vi "Calculate Place points.vi"(8 "error in (no error)":errorcluster, 11 "Control in":refnum<class "Control.lvclass">) -> (0 "error out":errorcluster, 3 "Control out":refnum<class "Control.lvclass">)   [LabVIEW 2012, in "Control.lvclass"]
uses:
  Control.lvclass
  Control.lvclass/Control.ctl
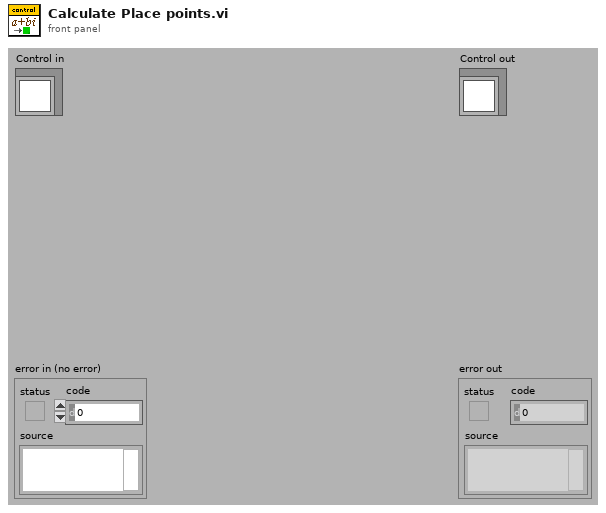
[diagram p1: front panel]
types:
  T1 = enum16{"User-specified Font", "Application Font", "System Font", "Dialog Font"}
  T2 = typedef "Control.lvclass/BX.Orientation__LCR _Modified.ctl" = u8
  T3 = typedef "Control.lvclass/_ui_tools_font.ctl" = cluster{"Font Name:":string, "Size":i16, "Strikeout?":bool, "Italic?":bool, "Underline?":bool, "Outline?":bool, "Shadow?":bool, "Bold?":bool}
  T4 = cluster{"left":i16, "top":i16, "right":i16, "bottom":i16}
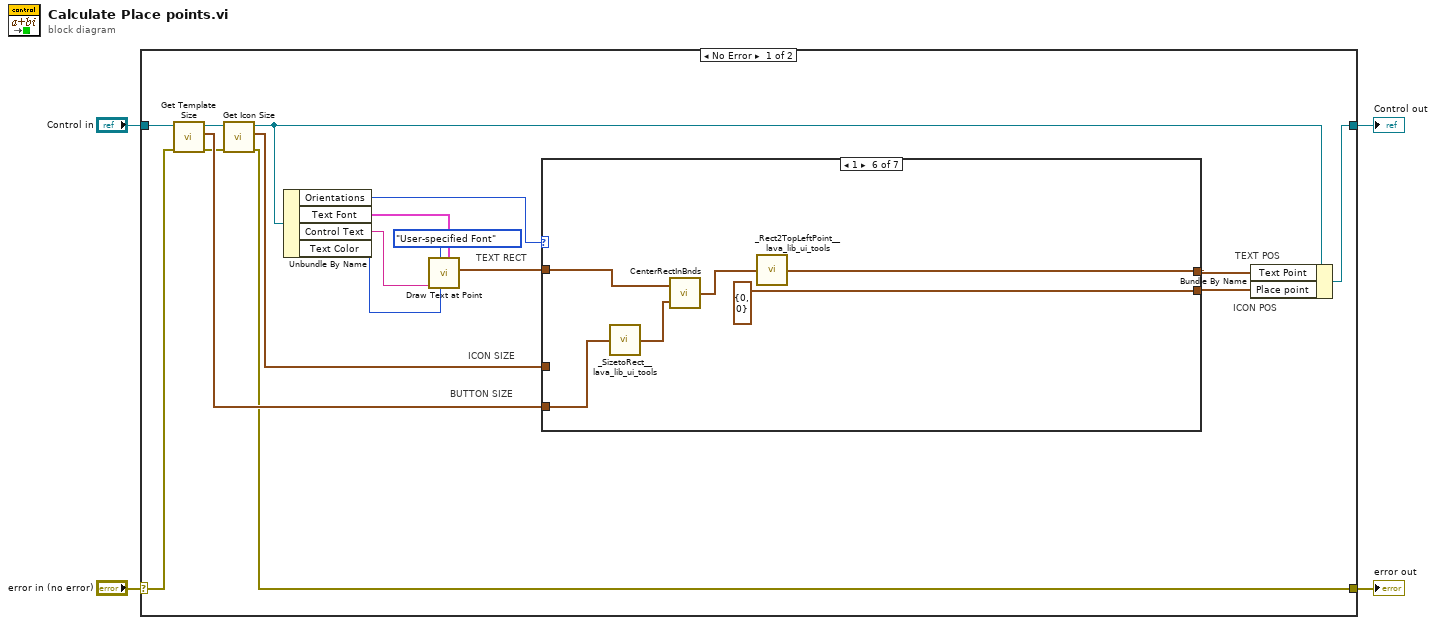
[diagram p0: block diagram]
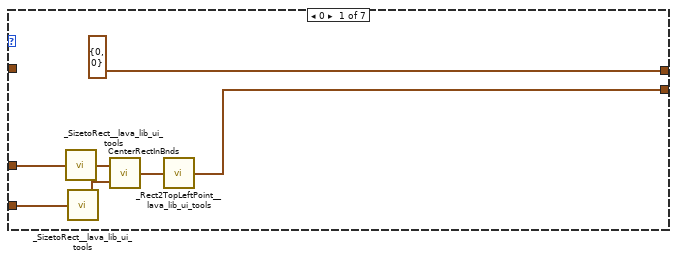
[diagram p2: hidden frame]
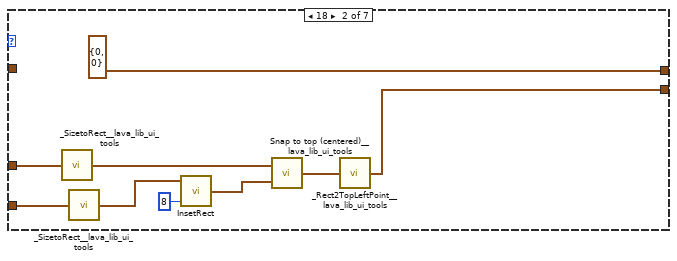
[diagram p3: hidden frame]
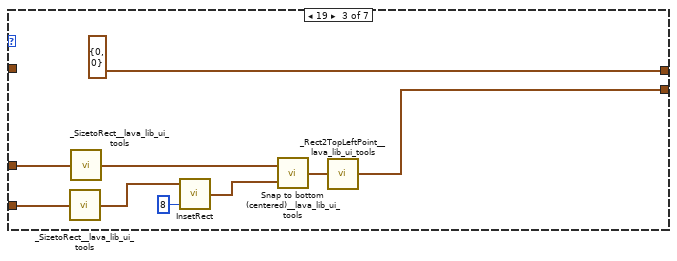
[diagram p4: hidden frame]
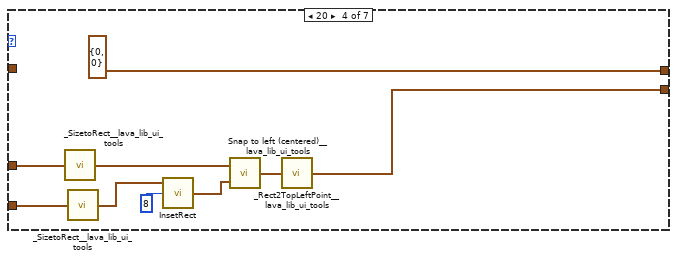
[diagram p5: hidden frame]
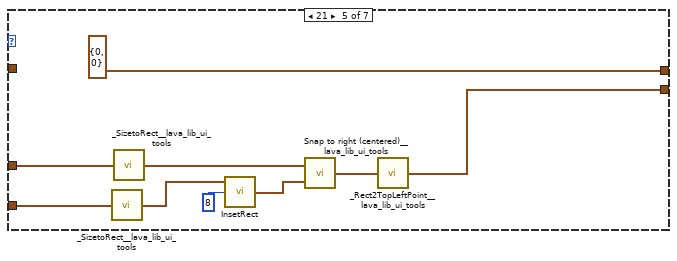
[diagram p6: hidden frame]
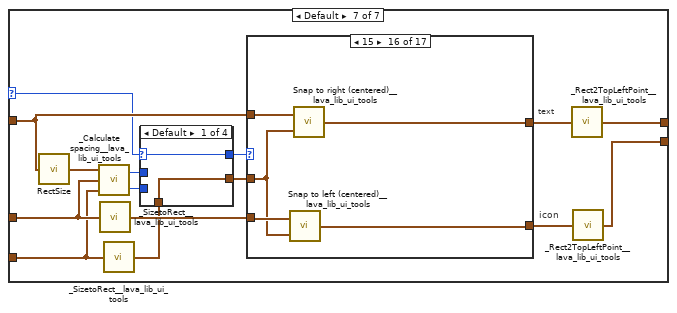
[diagram p7: hidden frame]
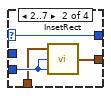
[diagram p8: hidden frame]
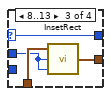
[diagram p9: hidden frame]
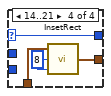
[diagram p10: hidden frame]
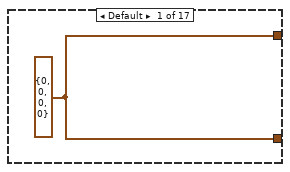
[diagram p11: hidden frame]
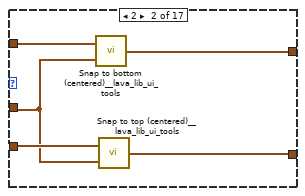
[diagram p12: hidden frame]
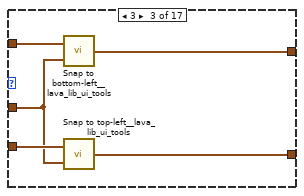
[diagram p13: hidden frame]
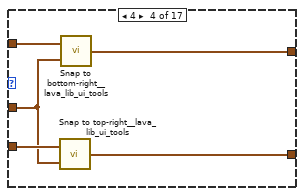
[diagram p14: hidden frame]
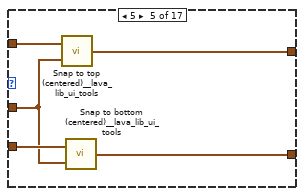
[diagram p15: hidden frame]
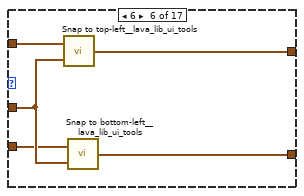
[diagram p16: hidden frame]
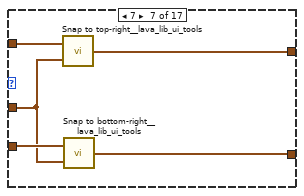
[diagram p17: hidden frame]
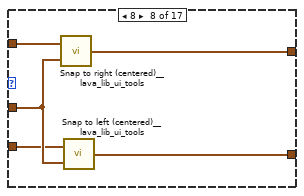
[diagram p18: hidden frame]
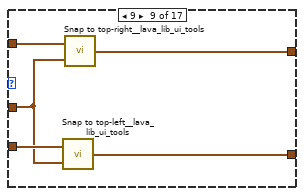
[diagram p19: hidden frame]
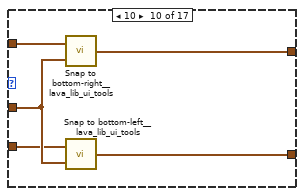
[diagram p20: hidden frame]
diagram:
  n1 = case shown="No Error" "error in (no error)" {
    selector: "error in (no error)" -> [w15 w197]
    tunnel: [w6 w197] -> w3
    tunnel: [w9 w196] -> w1
    tunnel: "Control in" -> [w14 w196]
    frame No Error {
      # "TEXT RECT"
      # "ICON SIZE"
      # "BUTTON SIZE"
      # "TEXT POS"
      # "ICON POS"
      n2 = call-dynamic "Get Template Size.vi"("error in (no error)"=w15, "Control in"=w14) -> ("error out"=w16:errorcluster, "Button Size"=w18:cluster{"Width":i32, "Height":i32}, "Control out"=w21:refnum<class "Control.lvclass">)  [unwired: 7 out]
      n3 = call-dynamic "Get Icon Size.vi"("error in (no error)"=w16, "Control in"=w21) -> ("error out"=w6:errorcluster, "Icon Size"=w19:cluster{"Width":i32, "Height":i32}, "Control out"=w10:refnum<class "Control.lvclass">)  [unwired: 7 out]
      n4 = Unbundle By Name(w10) -> ("Orientations"=w11:T2, "Text Font"=w12:T3, "Control Text"=w13:string, "Text Color"=w5:u32)
      n5 = call <vilib>:"Draw Text at Point.vi"("[user-specified font]"=w12, "text color(black)"=w5, "desired font(Application)"=T1."User-specified Font", "text"=w13) -> ("text rect"=w17:T4)  [unwired: 5 in, 2 out]
      n6 = case shown="1" w11 {
        selector: w11 -> [_ _ _ _ _ _ w75]
        tunnel: [cluster{"x":i32, "y":i32} {"x"=0, "y"=0} ("Point") cluster{"x":i32, "y":i32} {"x"=0, "y"=0} ("Point") cluster{"x":i32, "y":i32} {"x"=0, "y"=0} ("Point") cluster{"x":i32, "y":i32} {"x"=0, "y"=0} ("Point") cluster{"x":i32, "y":i32} {"x"=0, "y"=0} ("Point") w65 w85] -> w8
        tunnel: [w22 w32 w41 w50 w57 cluster{"x":i32, "y":i32} {"x"=0, "y"=0} ("Point") w82] -> w7
        tunnel: w18 -> [w26 w33 w43 w48 w61 w68 w72]
        tunnel: w17 -> [_ _ _ _ _ w70 w78]
        tunnel: w19 -> [w24 w35 w44 w52 w62 _ w83]
        frame 0 {
          n7 = call <vilib>:"_SizetoRect__lava_lib_ui_tools.vi"("size"=w24) -> ("bounds"=w25:T4)  [unwired: 4 out]
          n8 = call <vilib>:"_SizetoRect__lava_lib_ui_tools.vi"("size"=w26) -> ("bounds"=w27:T4)  [unwired: 4 out]
          n9 = call <vilib>:"CenterRectInBnds.vi"("bounds"=w27, "rect"=w25) -> ("centered rect"=w23:T4)
          n10 = call <vilib>:"_Rect2TopLeftPoint__lava_lib_ui_tools.vi"("bounds"=w23) -> ("TopLeft point"=w22:cluster{"x":i32, "y":i32})  [unwired: 4 out]
        }
        frame 18 {
          n11 = call <vilib>:"_SizetoRect__lava_lib_ui_tools.vi"("size"=w35) -> ("bounds"=w31:T4)  [unwired: 4 out]
          n12 = call <vilib>:"_SizetoRect__lava_lib_ui_tools.vi"("size"=w33) -> ("bounds"=w34:T4)  [unwired: 4 out]
          n13 = call <vilib>:"InsetRect.vi"("dv"=i16 8 ("dh"), "rect"=w34) -> ("inset rect"=w30:T4)  [unwired: 1 in]
          n14 = call <vilib>:"Snap to top (centered)__lava_lib_ui_tools.vi"("Large Rect"=w30, "Small Rect"=w31) -> ("Snapped to top center"=w29:T4)
          n15 = call <vilib>:"_Rect2TopLeftPoint__lava_lib_ui_tools.vi"("bounds"=w29) -> ("TopLeft point"=w32:cluster{"x":i32, "y":i32})  [unwired: 4 out]
        }
        frame 19 {
          n16 = call <vilib>:"_SizetoRect__lava_lib_ui_tools.vi"("size"=w43) -> ("bounds"=w42:T4)  [unwired: 4 out]
          n17 = call <vilib>:"_SizetoRect__lava_lib_ui_tools.vi"("size"=w44) -> ("bounds"=w40:T4)  [unwired: 4 out]
          n18 = call <vilib>:"InsetRect.vi"("dv"=i16 8 ("dh"), "rect"=w42) -> ("inset rect"=w39:T4)  [unwired: 1 in]
          n19 = call <vilib>:"Snap to bottom (centered)__lava_lib_ui_tools.vi"("Large Rect"=w39, "Small Rect"=w40) -> ("Snapped to bottom center"=w38:T4)
          n20 = call <vilib>:"_Rect2TopLeftPoint__lava_lib_ui_tools.vi"("bounds"=w38) -> ("TopLeft point"=w41:cluster{"x":i32, "y":i32})  [unwired: 4 out]
        }
        frame 20 {
          n21 = call <vilib>:"_SizetoRect__lava_lib_ui_tools.vi"("size"=w52) -> ("bounds"=w53:T4)  [unwired: 4 out]
          n22 = call <vilib>:"_SizetoRect__lava_lib_ui_tools.vi"("size"=w48) -> ("bounds"=w47:T4)  [unwired: 4 out]
          n23 = call <vilib>:"InsetRect.vi"("dh"=i16 8, "rect"=w47) -> ("inset rect"=w49:T4)  [unwired: 1 in]
          n24 = call <vilib>:"Snap to left (centered)__lava_lib_ui_tools.vi"("Large Rect"=w49, "Small Rect"=w53) -> ("Snapped to left center"=w51:T4)
          n25 = call <vilib>:"_Rect2TopLeftPoint__lava_lib_ui_tools.vi"("bounds"=w51) -> ("TopLeft point"=w50:cluster{"x":i32, "y":i32})  [unwired: 4 out]
        }
        frame 21 {
          n26 = call <vilib>:"_SizetoRect__lava_lib_ui_tools.vi"("size"=w61) -> ("bounds"=w60:T4)  [unwired: 4 out]
          n27 = call <vilib>:"_SizetoRect__lava_lib_ui_tools.vi"("size"=w62) -> ("bounds"=w59:T4)  [unwired: 4 out]
          n28 = call <vilib>:"InsetRect.vi"("dh"=i16 8, "rect"=w60) -> ("inset rect"=w58:T4)  [unwired: 1 in]
          n29 = call <vilib>:"Snap to right (centered)__lava_lib_ui_tools.vi"("Large Rect"=w58, "Small Rect"=w59) -> ("Snapped to right center"=w56:T4)
          n30 = call <vilib>:"_Rect2TopLeftPoint__lava_lib_ui_tools.vi"("bounds"=w56) -> ("TopLeft point"=w57:cluster{"x":i32, "y":i32})  [unwired: 4 out]
        }
        frame 1 {
          n31 = call <vilib>:"_SizetoRect__lava_lib_ui_tools.vi"("size"=w68) -> ("bounds"=w67:T4)  [unwired: 4 out]
          n32 = call <vilib>:"CenterRectInBnds.vi"("bounds"=w67, "rect"=w70) -> ("centered rect"=w66:T4)
          n33 = call <vilib>:"_Rect2TopLeftPoint__lava_lib_ui_tools.vi"("bounds"=w66) -> ("TopLeft point"=w65:cluster{"x":i32, "y":i32})  [unwired: 4 out]
        }
        frame Default {
          # "icon"
          # "text"
          n34 = call <vilib>:"RectSize.vi"("rect"=w78) -> ("point"=w84:cluster{"x":i16, "y":i16})
          n35 = call <vilib>:"_Calculate spacing__lava_lib_ui_tools.vi"("Button Size"=w72, "Icon Size"=w83, "Text Size"=w84) -> ("Vert. spacing"=w81:i32, "Horiz. spacing"=w74:i32)
          n36 = call <vilib>:"_SizetoRect__lava_lib_ui_tools.vi"("size"=w83) -> ("bounds"=w80:T4)  [unwired: 4 out]
          n37 = call <vilib>:"_SizetoRect__lava_lib_ui_tools.vi"("size"=w72) -> ("bounds"=w71:T4)  [unwired: 4 out]
          n38 = case shown="Default" w75 {
            selector: w75 -> [w86 w88 w92 w97]
            tunnel: w81 -> [_ w91 _ _]
            tunnel: [w87 w90 w95 w99] -> w77
            tunnel: w71 -> [w87 w89 w94 w98]
            tunnel: w74 -> [_ _ w93 _]
            tunnel: [w86 w88 w92 w97] -> w73
            frame Default {
            }
            frame 2..7 {
              n39 = call <vilib>:"InsetRect.vi"("dv"=w91, "dh"=w91, "rect"=w89) -> ("inset rect"=w90:T4)
            }
            frame 8..13 {
              n40 = call <vilib>:"InsetRect.vi"("dv"=w93, "dh"=w93, "rect"=w94) -> ("inset rect"=w95:T4)
            }
            frame 14..21 {
              w96 = i16 8 ("dh")
              n41 = call <vilib>:"InsetRect.vi"("dv"=w96, "dh"=w96, "rect"=w98) -> ("inset rect"=w99:T4)
            }
          }
          n42 = case shown="15" w73 {
            tunnel: w80 -> [_ w103 w108 w115 w119 w123 w128 w132 w139 w142 w148 w154 w157 w172 w178 w190 w192]
            tunnel: [w100 w101 w106 w114 w120 w122 w129 w131 w136 w141 w146 w155 w158 w167 w177 w189 w193] -> w79
            tunnel: w78 -> [_ w105 w110 w112 w118 w125 w126 w135 w140 w144 w150 w153 w159 w171 w176 w188 w195]
            tunnel: w77 -> [_ w102 w107 w113 w117 w124 w127 w133 w138 w145 w147 w152 w156 w170 w175 w187 w191]
            tunnel: [w100 w104 w109 w111 w116 w121 w130 w134 w137 w143 w149 w151 w160 w168 w185 w186 w194] -> w76
            frame Default {
              w100 = T4 {"left"=0, "top"=0, "right"=0, "bottom"=0} ("Snapped to bottom left")
            }
            frame 2 {
              n43 = call <vilib>:"Snap to bottom (centered)__lava_lib_ui_tools.vi"("Large Rect"=w102, "Small Rect"=w105) -> ("Snapped to bottom center"=w104:T4)
              n44 = call <vilib>:"Snap to top (centered)__lava_lib_ui_tools.vi"("Large Rect"=w102, "Small Rect"=w103) -> ("Snapped to top center"=w101:T4)
            }
            frame 3 {
              n45 = call <vilib>:"Snap to bottom-left__lava_lib_ui_tools.vi"("Fixed Rect"=w107, "Rect"=w110) -> ("Snapped to bottom left"=w109:T4)
              n46 = call <vilib>:"Snap to top-left__lava_lib_ui_tools.vi"("Fixed Rect"=w107, "Rect"=w108) -> ("Snapped to top left"=w106:T4)
            }
            frame 4 {
              n47 = call <vilib>:"Snap to top-right__lava_lib_ui_tools.vi"("Fixed Rect"=w113, "Rect"=w115) -> ("Snapped to top left"=w114:T4)
              n48 = call <vilib>:"Snap to bottom-right__lava_lib_ui_tools.vi"("Fixed Rect"=w113, "Rect"=w112) -> ("Snapped to bottom right"=w111:T4)
            }
            frame 5 {
              n49 = call <vilib>:"Snap to top (centered)__lava_lib_ui_tools.vi"("Large Rect"=w117, "Small Rect"=w118) -> ("Snapped to top center"=w116:T4)
              n50 = call <vilib>:"Snap to bottom (centered)__lava_lib_ui_tools.vi"("Large Rect"=w117, "Small Rect"=w119) -> ("Snapped to bottom center"=w120:T4)
            }
            frame 6 {
              n51 = call <vilib>:"Snap to top-left__lava_lib_ui_tools.vi"("Fixed Rect"=w124, "Rect"=w125) -> ("Snapped to top left"=w121:T4)
              n52 = call <vilib>:"Snap to bottom-left__lava_lib_ui_tools.vi"("Fixed Rect"=w124, "Rect"=w123) -> ("Snapped to bottom left"=w122:T4)
            }
            frame 7 {
              n53 = call <vilib>:"Snap to top-right__lava_lib_ui_tools.vi"("Fixed Rect"=w127, "Rect"=w126) -> ("Snapped to top left"=w130:T4)
              n54 = call <vilib>:"Snap to bottom-right__lava_lib_ui_tools.vi"("Fixed Rect"=w127, "Rect"=w128) -> ("Snapped to bottom right"=w129:T4)
            }
            frame 8 {
              n55 = call <vilib>:"Snap to right (centered)__lava_lib_ui_tools.vi"("Large Rect"=w133, "Small Rect"=w135) -> ("Snapped to right center"=w134:T4)
              n56 = call <vilib>:"Snap to left (centered)__lava_lib_ui_tools.vi"("Large Rect"=w133, "Small Rect"=w132) -> ("Snapped to left center"=w131:T4)
            }
            frame 9 {
              n57 = call <vilib>:"Snap to top-left__lava_lib_ui_tools.vi"("Fixed Rect"=w138, "Rect"=w139) -> ("Snapped to top left"=w136:T4)
              n58 = call <vilib>:"Snap to top-right__lava_lib_ui_tools.vi"("Fixed Rect"=w138, "Rect"=w140) -> ("Snapped to top left"=w137:T4)
            }
            frame 10 {
              n59 = call <vilib>:"Snap to bottom-right__lava_lib_ui_tools.vi"("Fixed Rect"=w145, "Rect"=w144) -> ("Snapped to bottom right"=w143:T4)
              n60 = call <vilib>:"Snap to bottom-left__lava_lib_ui_tools.vi"("Fixed Rect"=w145, "Rect"=w142) -> ("Snapped to bottom left"=w141:T4)
            }
            frame 11 {
              n61 = call <vilib>:"Snap to left (centered)__lava_lib_ui_tools.vi"("Large Rect"=w147, "Small Rect"=w150) -> ("Snapped to left center"=w149:T4)
              n62 = call <vilib>:"Snap to right (centered)__lava_lib_ui_tools.vi"("Large Rect"=w147, "Small Rect"=w148) -> ("Snapped to right center"=w146:T4)
            }
            frame 12 {
              n63 = call <vilib>:"Snap to top-right__lava_lib_ui_tools.vi"("Fixed Rect"=w152, "Rect"=w154) -> ("Snapped to top left"=w155:T4)
              n64 = call <vilib>:"Snap to top-left__lava_lib_ui_tools.vi"("Fixed Rect"=w152, "Rect"=w153) -> ("Snapped to top left"=w151:T4)
            }
            frame 13 {
              n65 = call <vilib>:"Snap to bottom-left__lava_lib_ui_tools.vi"("Fixed Rect"=w156, "Rect"=w159) -> ("Snapped to bottom left"=w160:T4)
              n66 = call <vilib>:"Snap to bottom-right__lava_lib_ui_tools.vi"("Fixed Rect"=w156, "Rect"=w157) -> ("Snapped to bottom right"=w158:T4)
            }
            frame 14 {
              n67 = call <vilib>:"Snap to left (centered)__lava_lib_ui_tools.vi"("Large Rect"=w170, "Small Rect"=w171) -> ("Snapped to left center"=w169:T4)
              n68 = call <vilib>:"Snap to left (centered)__lava_lib_ui_tools.vi"("Large Rect"=w170, "Small Rect"=w172) -> ("Snapped to left center"=w167:T4)
              n69 = call <vilib>:"RectSize.vi"("rect"=w167) -> ("point"=w166:cluster{"x":i16, "y":i16})
              n70 = Unbundle By Name(w166) -> ("x"=w165:i16)
              n71 = Add(x=w165, y=i16 12) -> (x+y=w161:i16)
              n72 = Bundle By Name(cluster=cluster{"x":i16, "y":i16} {"x"=0, "y"=0} ("point"), "x"=w161) -> (w162:cluster{"x":i16, "y":i16})
              n73 = call <vilib>:"POffsetRect.vi"("rect"=w169, "point"=w162) -> ("offset rect"=w168:T4)
            }
            frame 17 {
              n74 = call <vilib>:"Snap to right (centered)__lava_lib_ui_tools.vi"("Large Rect"=w175, "Small Rect"=w176) -> ("Snapped to right center"=w174:T4)
              n75 = call <vilib>:"Snap to right (centered)__lava_lib_ui_tools.vi"("Large Rect"=w175, "Small Rect"=w178) -> ("Snapped to right center"=w177:T4)
              n76 = call <vilib>:"RectSize.vi"("rect"=w177) -> ("point"=w184:cluster{"x":i16, "y":i16})
              n77 = Unbundle By Name(w184) -> ("x"=w183:i16)
              n78 = Add(x=w183, y=i16 12) -> (x+y=w179:i16)
              n79 = Negate(x=w179) -> (-x=w173:i16)
              n80 = Bundle By Name(cluster=cluster{"x":i16, "y":i16} {"x"=0, "y"=0} ("point"), "x"=w173) -> (w180:cluster{"x":i16, "y":i16})
              n81 = call <vilib>:"POffsetRect.vi"("rect"=w174, "point"=w180) -> ("offset rect"=w185:T4)
            }
            frame 15 {
              n82 = call <vilib>:"Snap to left (centered)__lava_lib_ui_tools.vi"("Large Rect"=w187, "Small Rect"=w190) -> ("Snapped to left center"=w189:T4)
              n83 = call <vilib>:"Snap to right (centered)__lava_lib_ui_tools.vi"("Large Rect"=w187, "Small Rect"=w188) -> ("Snapped to right center"=w186:T4)
            }
            frame 16 {
              n84 = call <vilib>:"Snap to left (centered)__lava_lib_ui_tools.vi"("Large Rect"=w191, "Small Rect"=w195) -> ("Snapped to left center"=w194:T4)
              n85 = call <vilib>:"Snap to right (centered)__lava_lib_ui_tools.vi"("Large Rect"=w191, "Small Rect"=w192) -> ("Snapped to right center"=w193:T4)
            }
          }
          n86 = call <vilib>:"_Rect2TopLeftPoint__lava_lib_ui_tools.vi"("bounds"=w76) -> ("TopLeft point"=w85:cluster{"x":i32, "y":i32})  [unwired: 4 out]
          n87 = call <vilib>:"_Rect2TopLeftPoint__lava_lib_ui_tools.vi"("bounds"=w79) -> ("TopLeft point"=w82:cluster{"x":i32, "y":i32})  [unwired: 4 out]
        }
      }
      n88 = Bundle By Name(cluster=w10, "Text Point"=w8, "Place point"=w7) -> (w9:refnum<class "Control.lvclass">)
    }
    frame Error {
    }
  }
  "error out" <- w3
  "Control out" <- w1
